vi "Respond to Command.vi"(6 "timeout (-1 ms)":i32=-1, 8 "error in (no error)":errorcluster, 9 "message value":string, 10 "ResponseInfo":T1, 11 "VeriStand Comm in":refnum<class "VeriStand Comm.lvclass">) -> (0 "error out":errorcluster, 1 "Written?":bool, 3 "VeriStand Comm out":refnum<class "VeriStand Comm.lvclass">)   [LabVIEW 2018, in "NI VeriStand Addon Network Comm.lvlib" / "VeriStand Comm.lvclass"]
uses:
  VeriStand Comm.lvclass
  _Types/Response Information.ctl
  <vilib>/NI/AMC/Create Single Message.vi
  <vilib>/NI/AMC/Update Message Routing Info.vi
  <vilib>/NI/AMC/Send Message.vi
  <vilib>/NI/AMC/AMC.lvlib
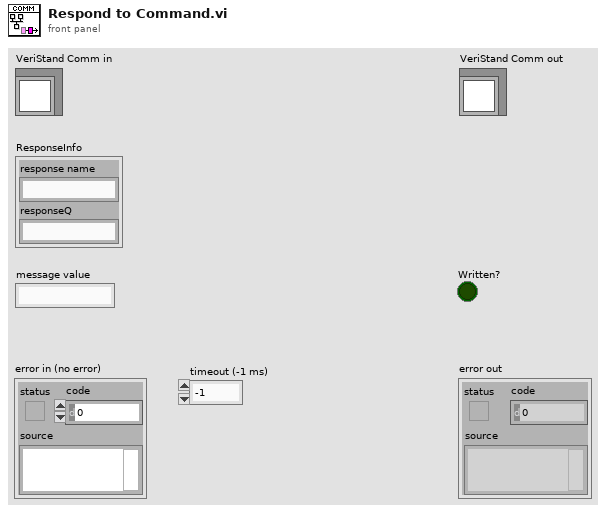
[diagram p1: front panel]
types:
  T1 = typedef "NI VeriStand Addon Network Comm.lvlib/VeriStand Comm.lvclass/Response Information.ctl" = cluster{"response name":string, "responseQ":string}
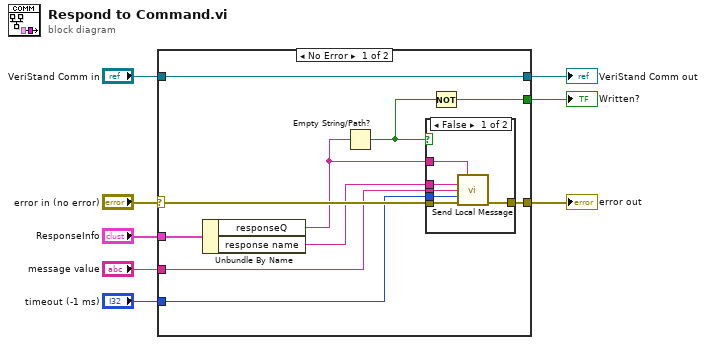
[diagram p0: block diagram]
diagram:
  n1 = case shown="No Error" "error in (no error)" {
    selector: "error in (no error)" -> [w16 w27]
    tunnel: [w17 w27] -> w7
    tunnel: [w18 w26] -> w5
    tunnel: "VeriStand Comm in" -> [w18 w26]
    tunnel: "message value" -> [w15 _]
    tunnel: "timeout (-1 ms)" -> [w14 _]
    tunnel: "ResponseInfo" -> [w13 _]
    tunnel: [w9 _] -> w1
    frame No Error {
      n2 = Unbundle By Name(w13) -> ("responseQ"=w11:string, "response name"=w12:string)
      n3 = Empty String/Path?(string/path=w11) -> (empty?=w10:bool)
      n4 = case shown="False" w10 {
        tunnel: [w24 w25] -> w17
        tunnel: w16 -> [w23 w25]
        tunnel: w15 -> [w22 _]
        tunnel: w14 -> [w21 _]
        tunnel: w12 -> [w20 _]
        tunnel: w11 -> [w19 _]
        frame False {
          n5 = call <vilib>:"Send Local Message.vi"("receiver process (\"\" - local)"=w19, "message name"=w20, "message value"=w22, "timeout (-1 ms)"=w21, "error in"=w23) -> ("error out"=w24:errorcluster)  [unwired: 8 in, 2 out]
        }
        frame True {
        }
      }
      n6 = Not(x=w10) -> (.not. x?=w9:bool)
    }
    frame Error {
    }
  }
  "error out" <- w7
  "VeriStand Comm out" <- w5
  "Written?" <- w1
